vi "TestTicklishSerial.vi"() -> ()   [LabVIEW 2015]
panel:
  in  "Pulse Number 2":i32
  in  "Pulse Interval 2":dbl
  in  "Pulse Length 2":dbl
  in  "Number 2":i32
  in  "Interval 2":dbl
  in  "Delay 2":dbl
  out "time-sync":T1
  in  "Pulse Number":i32
  in  "Pulse Interval":dbl
  in  "Pulse Length":dbl
  in  "Number":i32
  in  "Interval":dbl
  in  "Delay":dbl
  in  "Channel":T2(ring)
  in  "Run Stim":bool
  in  "Sync?":bool
  in  "Fixed-length response":bool
  out "error out":errorcluster
  out "Result string":string
  out "Serial USB port name out":refnum<visa-resource-name>
  in  "byte count":u32
  in  "write buffer":string
  in  "Serial USB Stimulus Port":refnum<visa-resource-name>="COM4"
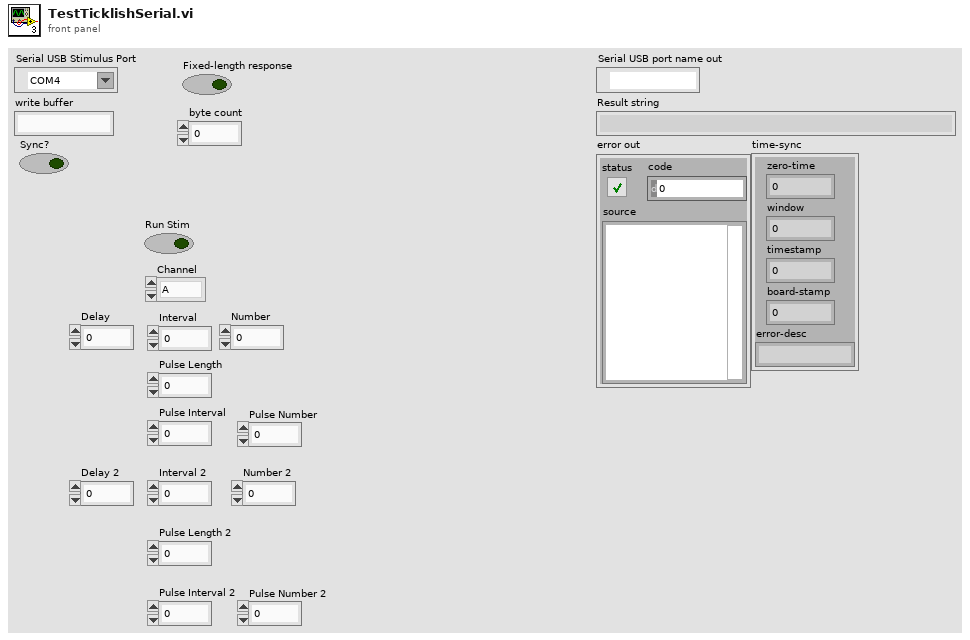
[diagram p1: front panel]
types:
  T1 = cluster{"zero-time":dbl, "window":dbl, "timestamp":dbl, "board-stamp":dbl, "error-desc":string}
  T2 = enum16{"A", "B", "C", "D", "E", "F", "G", "H", "I", "J", "K", "L", "M", "N", "O", "P", "Q", "R", "S", "T", "U", "V", "W", "X"}
  T3 = cluster{"Channel":enum16{"A", "B", "C", "D", "E", "F", "G", "H", "I", "J", "K", "L", "M", "N", "O", "P", "Q", "R", "S", "T", "U", "V", "W", "X"}, "Delay":dbl, "Interval":dbl, "Number":i32, "Pulse Length":dbl, "Pulse Interval":dbl, "Pulse Number":i32}
  T4 = cluster{"Channel":enum16{"A", "B", "C", "D", "E", "F", "G", "H", "I", "J", "K", "L", "M", "N", "O", "P", "Q", "R", "S", "T", "U", "V", "W", "X"}, "Delay":dbl, "Interval":dbl, "Number":i32, "Pulse Length":dbl, "Pulse Interval":dbl, "Pulse Number":i32}[]
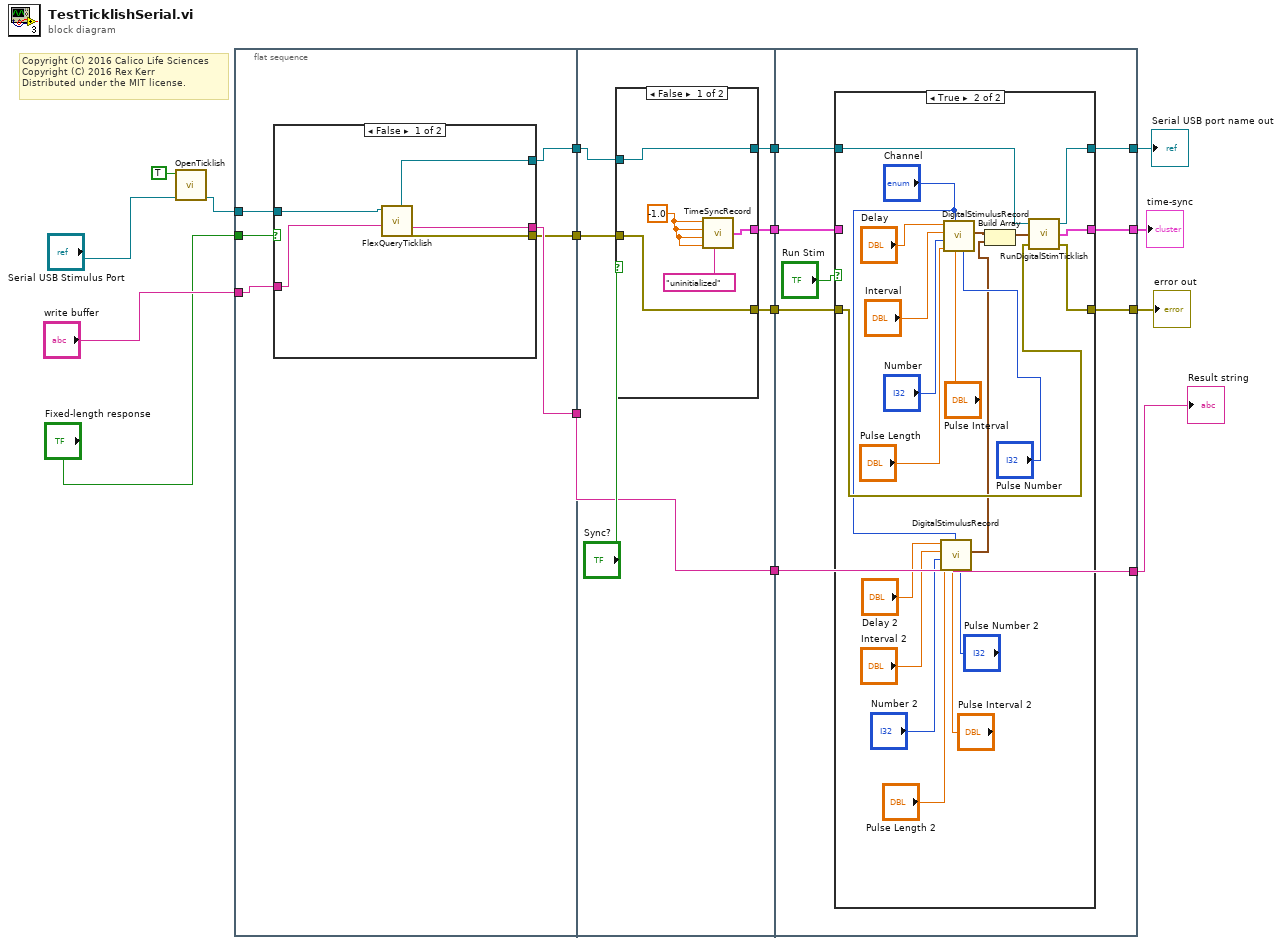
[diagram p0: block diagram]
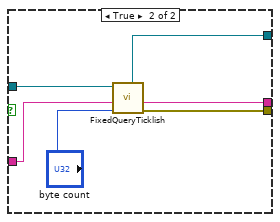
[diagram p2: hidden frame]
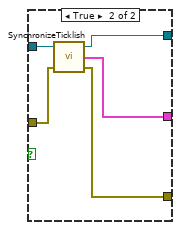
[diagram p3: hidden frame]
diagram:
  # "Copyright (C) 2016 Calico Life Sciences\nCopyright (C) 2016 Rex Kerr\nDistributed under the MIT license."
  n1 = call "OpenTicklish.vi"("Serial USB Stimulus Port"="Serial USB Stimulus Port", "Use Serial USB Stimulus"=TRUE) -> ("VISA resource name out"=w14:refnum<visa-resource-name>)  [unwired: 9 in]
  n2 = flat-sequence {
    tunnel: w14 -> [w22]
    tunnel: "write buffer" -> [w21]
    tunnel: "Fixed-length response" -> [w20]
    tunnel: [w19] -> w9
    tunnel: [w18] -> w8
    tunnel: [w17] -> w6
    tunnel: w9 -> [w37]
    tunnel: w8 -> [w34]
    tunnel: w6 -> [w40]
    tunnel: [w36] -> w5
    tunnel: [w38] -> w4
    tunnel: [w39] -> w3
    tunnel: [w34] -> w2
    tunnel: [w58] -> w7
    tunnel: [w51] -> w10
    tunnel: [w53] -> w1
    tunnel: [w55] -> w11
    tunnel: w5 -> [w56]
    tunnel: w4 -> [w54]
    tunnel: w3 -> [w52]
    tunnel: w2 -> [w58]
    frame #0 {
      n3 = case shown="False" w20 {
        tunnel: w22 -> [w27 w33]
        tunnel: [w25 w31] -> w19
        tunnel: [w24 w30] -> w18
        tunnel: [w23 w29] -> w17
        tunnel: w21 -> [w26 w28]
        frame False {
          n4 = call "FlexQueryTicklish.vi"("write buffer"=w26, "Serial USB port name"=w27) -> ("error out"=w23:errorcluster, "Result string"=w24:string, "Serial USB port name out"=w25:refnum<visa-resource-name>)  [unwired: 7 in]
        }
        frame True {
          n5 = call "FixedQueryTicklish.vi"("byte count"="byte count", "write buffer"=w28, "Serial USB port name"=w33) -> ("error out"=w29:errorcluster, "Result string"=w30:string, "Serial USB port name out"=w31:refnum<visa-resource-name>)  [unwired: 6 in]
        }
      }
    }
    frame #1 {
      n6 = case shown="False" "Sync?" {
        tunnel: w40 -> [w44 w50]
        tunnel: [w44 w49] -> w39
        tunnel: [w43 w48] -> w38
        tunnel: w37 -> [w45 w47]
        tunnel: [w45 w46] -> w36
        frame False {
          w42 = -1.0 ("zero-time")
          n7 = call "TimeSyncRecord.vi"("zero-time"=w42, "window"=w42, "timestamp"=w42, "error-desc"="uninitialized", "board-stamp"=w42) -> ("output cluster"=w43:T1)  [unwired: 3 in]
        }
        frame True {
          n8 = call "SynchronizeTicklish.vi"("error in (no error)"=w50, "Serial USB port name"=w47) -> ("error out"=w49:errorcluster, "time-sync"=w48:T1, "Serial USB port name out"=w46:refnum<visa-resource-name>)  [unwired: 1 in]
        }
      }
    }
    frame #2 {
      n9 = case shown="True" "Run Stim" {
        tunnel: w56 -> [w61 w82]
        tunnel: [w61 w81] -> w55
        tunnel: w54 -> [w60 _]
        tunnel: [w60 w79] -> w53
        tunnel: w52 -> [w59 w71]
        tunnel: [w59 w80] -> w51
        frame False {
        }
        frame True {
          n10 = call "DigitalStimulusRecord.vi"("Pulse Number"="Pulse Number 2", "Pulse Interval"="Pulse Interval 2", "Channel"="Channel", "Pulse Length"="Pulse Length 2", "Number"="Number 2", "Interval"="Interval 2", "Delay"="Delay 2") -> ("digital stimulus"=w69:T3)  [unwired: 4 in]
          n11 = call "DigitalStimulusRecord.vi"("Pulse Number"="Pulse Number", "Pulse Interval"="Pulse Interval", "Channel"="Channel", "Pulse Length"="Pulse Length", "Number"="Number", "Interval"="Interval", "Delay"="Delay") -> ("digital stimulus"=w78:T3)  [unwired: 4 in]
          n12 = Build Array(w78, w69) -> (w77:T4)
          n13 = call "RunDigitalStimTicklish.vi"("error in (no error)"=w71, "digital stimuli"=w77, "Serial USB port name"=w82) -> ("error out"=w80:errorcluster, "time-sync"=w79:T1, "Serial USB port name out"=w81:refnum<visa-resource-name>)
        }
      }
    }
  }
  "Serial USB port name out" <- w11
  "error out" <- w10
  "Result string" <- w7
  "time-sync" <- w1
